vi "Pump Tags.vi"(11 "Pump Module Configs":T1[](array[typedef]) {"Settings"."Ismatech 3 Channel Settings"."Channel Number" min=0 max=3; "Settings"."Ismatech 3 Channel Settings"."Pump Number" min=1; "Settings"."ASIA Pump C"."channel" min=0 max=1 step=1; "Settings"."Masterflex"."Pump Number" min=1.0 max=20.0 step=1.0; "Settings"."Ismatech"."Pump Number" min=1.0 max=20.0 step=1.0}) -> (1 "Pump Module Tag Names":T15, 2 "All Boolean Tags 3":string[](array[string]), 3 "All  Numeric Tags 3":string[](array[string]), 4 "Pump Module Tags Array":T15[](array[typedef]))   [LabVIEW 2018]
uses:
  Pump Module Folder/Pump Module Tag Names Cluster.ctl
  Pump Module Folder/Pump Module Config Cluster.ctl
  <vilib>/Utility/miscctls.llb/LVPoint32TypeDef.ctl
  Pump Module Folder/Pump Module Settings Cluster.ctl
  Measure Instrument/PID 2 Output Enum.ctl
  Ismatec ISM 831C/Controls/Ismatech ISM831C Settings Cluster.ctl
  Ismatec 78001/Ismatec 4083.ctl
  Masterflex 7550-30/Controls/Settings Cluster.ctl
  VICI M50 Party Mode/Settings Cluster.ctl
  Tacmina QI/Tacmina QI DAQ Setting.ctl
  KNF Pump/Settings Cluster plus SIMDOS.ctl
  ASIA Pump/Pump Settings.ctl
  FLOM Pump/Settings Cluster.ctl
  SSI PR Class/SSI PR or LD Settings Cluster.ctl
  Masterflex 75211/Masterflex 75211 DAQ Setting.ctl
  Pump Module Folder/Pump Module.lvlib
  Ismatec ISM 831C/Ismatec ISM 831C.lvlib
  Masterflex 7550-30/Masterflex 7550-30.lvlib
  VICI M50 Party Mode/VICI M6 M50 Party Mode.lvlib
  Tacmina QI/Tacmina QI.lvlib
  KNF Pump/KNF SIMDOS.lvlib
  ASIA Pump.lvlib
  FLOM Pump/FLOM Pump.lvlib
  SSI PR Class/SSI PR or LD Pump.lvlib
  Masterflex 75211/Masterflex 75211.lvlib
  Ismatec 78001/Ismatec 4308.lvlib
panel:
  # "Output Instruments"
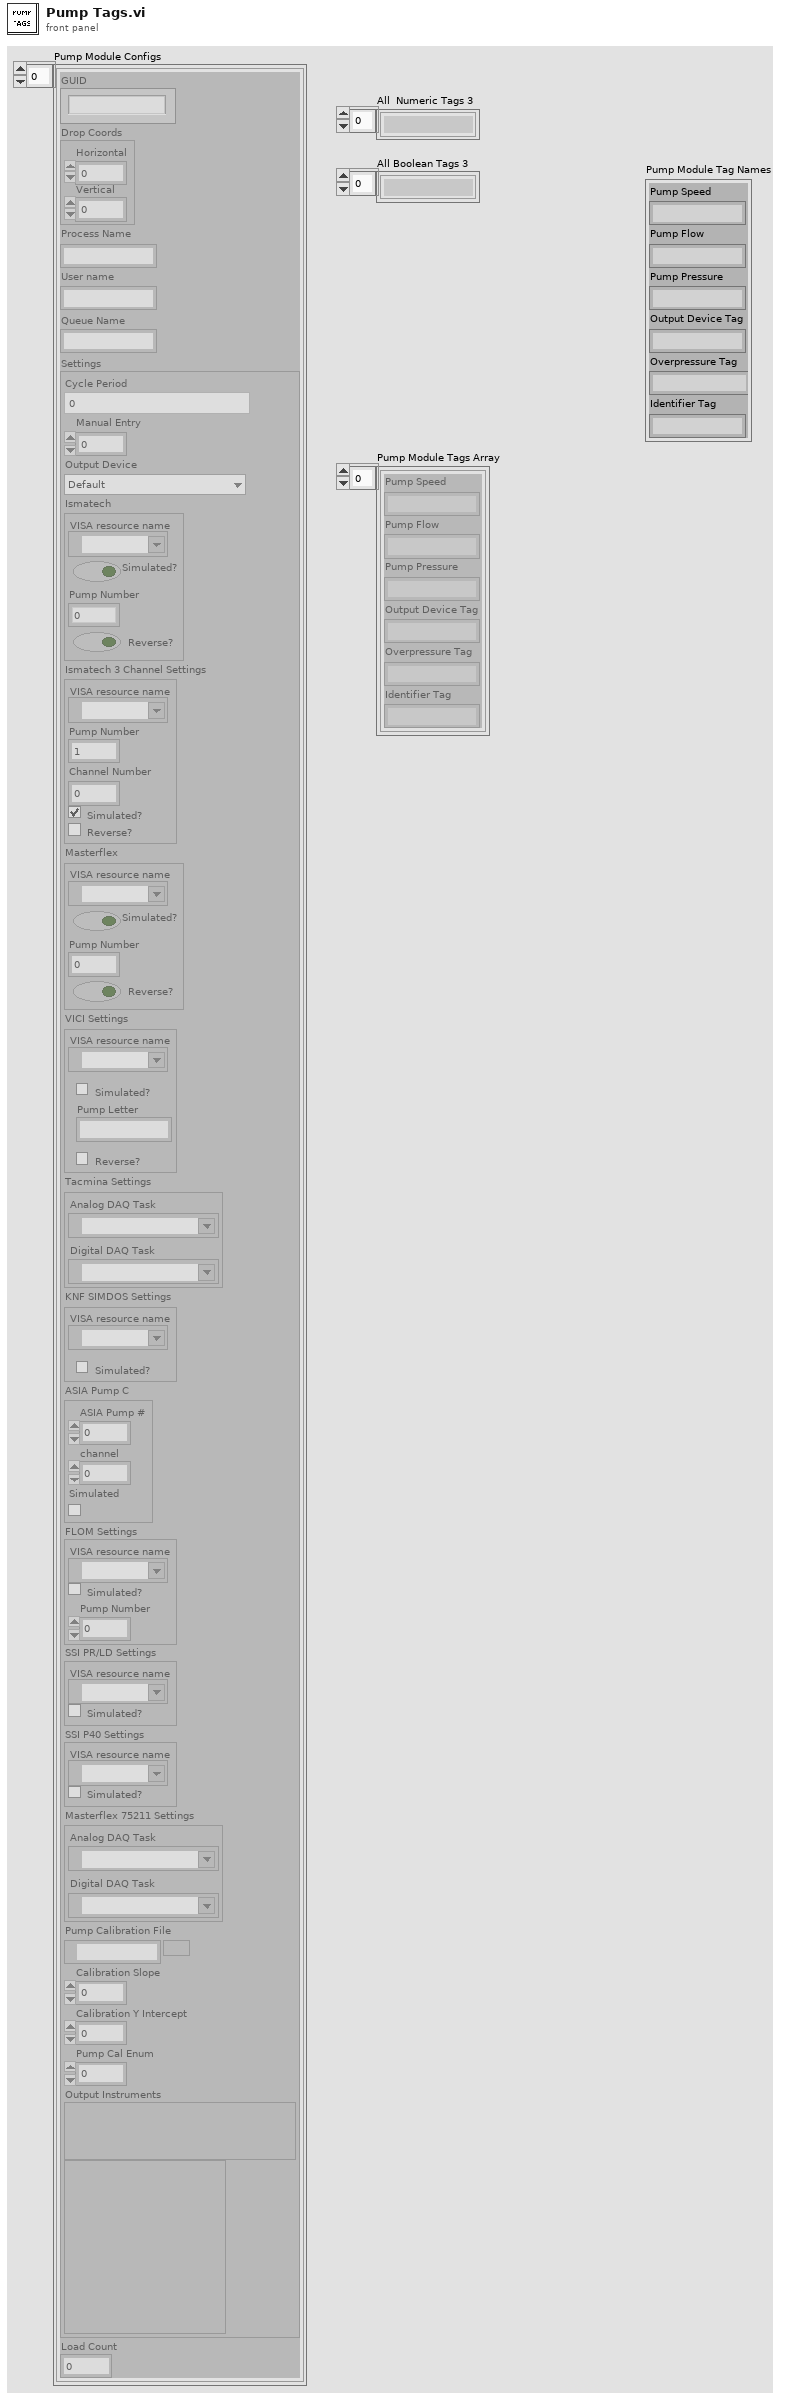
[diagram p1: front panel]
types:
  T1 = typedef "Pump Module.lvlib/Pump Module Config Cluster.ctl" = cluster{"GUID":string, "Drop Coords":T2, "Process Name":string, "User name":string, "Queue Name":string, "Settings":T3, "Load Count":i32}
  T2 = typedef "LVPoint32TypeDef.ctl" = cluster{"Horizontal":i32, "Vertical":i32}
  T3 = typedef "Pump Module.lvlib/Pump Module Settings Cluster.ctl" = cluster{"Cycle Period":dbl, "Manual Entry":dbl, "Output Device":T4, "Ismatech":T5, "Ismatech 3 Channel Settings":T6, "Masterflex":T7, "VICI Settings":T8, "Tacmina Settings":T9, "KNF SIMDOS Settings":T10, "ASIA Pump C":T11, "FLOM Settings":T12, "SSI PR/LD Settings":T13, "SSI P40 Settings":T13, "Masterflex 75211 Settings":T14, "Pump Calibration File":path, "Calibration Slope":dbl, "Calibration Y Intercept":dbl, "Pump Cal Enum":u16}
  T4 = typedef "PID 2 Output Enum.ctl" = enum16{"Default", "Ismatec ISM 4308", "Ismatec ISM 831C", "Masterflex 7550-30", "VICI", "Tacmina QI", "KNF SIMDOS", "ASIA Type C", "FLOM UI-22-11", "SSI PR/LD", "SSI P40", "Masterflex 75211-70"}
  T5 = typedef "Ismatec ISM 831C.lvlib/Ismatech ISM831C Settings Cluster.ctl" = cluster{"VISA resource name":refnum<visa-resource-name>, "Simulated?":bool, "Pump Number":dbl, "Reverse?":bool}
  T6 = typedef "Ismatec 4308.lvlib/Ismatec 4083.ctl" = cluster{"VISA resource name":refnum<visa-resource-name>, "Pump Number":i16, "Channel Number":i16, "Simulated?":bool, "Reverse?":bool}
  T7 = typedef "Masterflex 7550-30.lvlib/Settings Cluster.ctl" = cluster{"VISA resource name":refnum<visa-resource-name>, "Simulated?":bool, "Pump Number":dbl, "Reverse?":bool}
  T8 = typedef "VICI M6 M50 Party Mode.lvlib/Settings Cluster.ctl" = cluster{"VISA resource name":refnum<visa-resource-name>, "Simulated?":bool, "Pump Letter":string, "Reverse?":bool}
  T9 = typedef "Tacmina QI.lvlib/Tacmina QI DAQ Setting.ctl" = cluster{"Analog DAQ Task":refnum<k21>, "Digital DAQ Task":refnum<k21>}
  T10 = typedef "KNF SIMDOS.lvlib/Settings Cluster plus SIMDOS.ctl" = cluster{"VISA resource name":refnum<visa-resource-name>, "Simulated?":bool}
  T11 = typedef "ASIA Pump.lvlib/Pump Settings.ctl" = cluster{"ASIA Pump #":i32, "channel":i32, "Simulated":bool}
  T12 = typedef "FLOM Pump.lvlib/Settings Cluster.ctl" = cluster{"VISA resource name":refnum<visa-resource-name>, "Simulated?":bool, "Pump Number":dbl}
  T13 = typedef "SSI PR or LD Pump.lvlib/SSI PR or LD Settings Cluster.ctl" = cluster{"VISA resource name":refnum<visa-resource-name>, "Simulated?":bool}
  T14 = typedef "Masterflex 75211.lvlib/Masterflex 75211 DAQ Setting.ctl" = cluster{"Analog DAQ Task":refnum<k21>, "Digital DAQ Task":refnum<k21>}
  T15 = typedef "Pump Module.lvlib/Pump Module Tag Names Cluster.ctl" = cluster{"Pump Speed":string, "Pump Flow":string, "Pump Pressure":string, "Output Device Tag":string, "Overpressure Tag":string, "Identifier Tag":string}
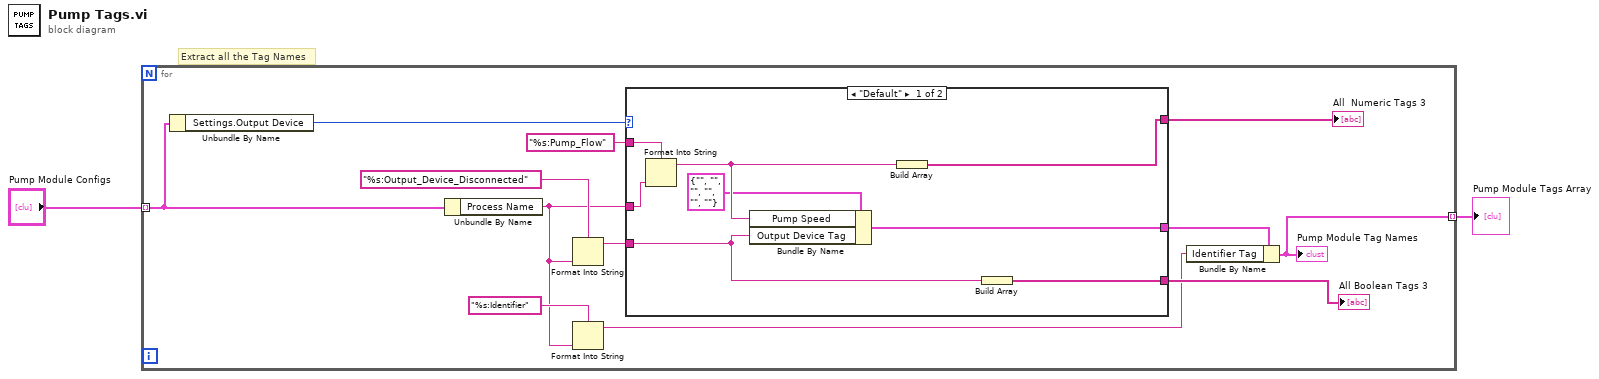
[diagram p0: block diagram]
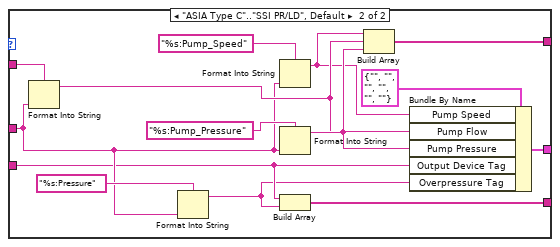
[diagram p2: hidden frame]
diagram:
  # "Extract all the Tag Names"
  n1 = for {
    tunnel: "Pump Module Configs" -> [w8] mode=indexing
    tunnel: [w4] -> w1 mode=indexing
    n2 = Unbundle By Name(w8) -> ("Settings.Output Device"=w13:T4)
    n3 = Unbundle By Name(w8) -> ("Process Name"=w6:string)
    n4 = Format Into String(format string="%s:Output_Device_Disconnected", w6) -> (resulting string=w10:string)  [unwired: 2 in, 1 out]
    n5 = Format Into String(format string="%s:Identifier", w6) -> (resulting string=w3:string)  [unwired: 2 in, 1 out]
    n6 = case shown="\"Default\"" w13 {
      tunnel: w6 -> [w21 w27]
      tunnel: w10 -> [w17 w26]
      tunnel: [w22 w31] -> w12
      tunnel: [w19 w30] -> w5
      tunnel: [w16 w25] -> w11
      tunnel: "%s:Pump_Flow" ("format string") -> [w15 w23]
      frame "Default" {
        n7 = Format Into String(format string=w15, w21) -> (resulting string=w20:string)  [unwired: 2 in, 1 out]
        n8 = Bundle By Name(cluster=T15 {"Pump Speed"="", "Pump Flow"="", "Pump Pressure"="", "Output Device Tag"="", "Overpressure Tag"="", "Identifier Tag"=""} ("Feed Module Tag Names"), "Pump Speed"=w20, "Output Device Tag"=w17) -> (w19:T15)
        n9 = Build Array(w20) -> (w22:string[])
        n10 = Build Array(w17) -> (w16:string[])
      }
      frame "ASIA Type C".."SSI PR/LD", Default {
        n11 = Format Into String(format string=w23, w27) -> (resulting string=w35:string)  [unwired: 2 in, 1 out]
        n12 = Format Into String(format string="%s:Pressure", w27) -> (resulting string=w24:string)  [unwired: 2 in, 1 out]
        n13 = Format Into String(format string="%s:Pump_Speed", w27) -> (resulting string=w29:string)  [unwired: 2 in, 1 out]
        n14 = Format Into String(format string="%s:Pump_Pressure", w27) -> (resulting string=w36:string)  [unwired: 2 in, 1 out]
        n15 = Build Array(w26, w24) -> (w25:string[])
        n16 = Build Array(w29, w35, w36) -> (w31:string[])
        n17 = Bundle By Name(cluster=T15 {"Pump Speed"="", "Pump Flow"="", "Pump Pressure"="", "Output Device Tag"="", "Overpressure Tag"="", "Identifier Tag"=""} ("Feed Module Tag Names"), "Pump Speed"=w29, "Pump Flow"=w35, "Pump Pressure"=w36, "Output Device Tag"=w26, "Overpressure Tag"=w24) -> (w30:T15)
      }
    }
    "All Boolean Tags 3" <- w11
    "All  Numeric Tags 3" <- w12
    n18 = Bundle By Name(cluster=w5, "Identifier Tag"=w3) -> (w4:T15)
    "Pump Module Tag Names" <- w4
  }
  "Pump Module Tags Array" <- w1
